vi "ManageQMess.vi"(8 "ErrorIn(No Error)":errorcluster caption="entrée d'erreur (pas d'erreur)", 10 "Message":string, 11 "AppliedMotionDrive.lvclass":refnum<class "AppliedMotionDrive.lvclass">) -> (0 "sortie d'erreur":errorcluster, 3 "AppliedMotionDrive.lvclass Out":refnum<class "AppliedMotionDrive.lvclass">)   [LabVIEW 2019, in "AppliedMotionDrive.lvclass"]
uses:
  AppliedMotionDrive.lvclass
  BaseDevice/ClassQueueMess.ctl
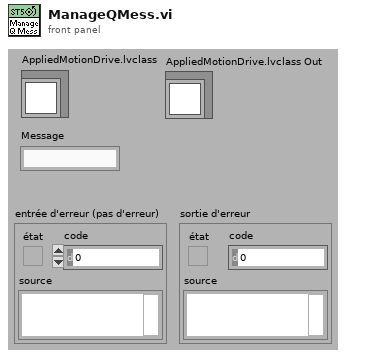
[diagram p1: front panel]
types:
  T1 = typedef "ClassQueueMess.ctl" = u16
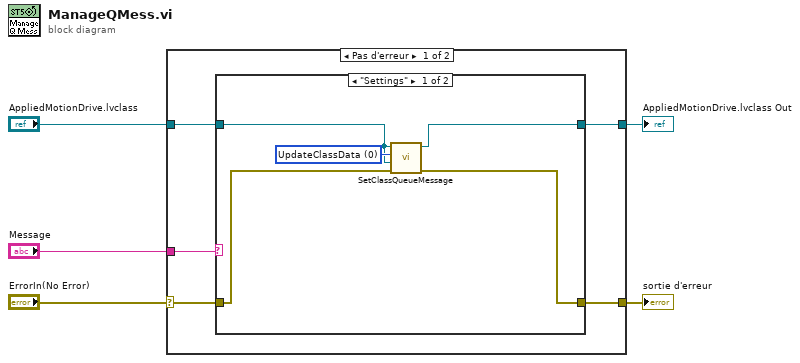
[diagram p0: block diagram]
diagram:
  n1 = case shown="Pas d'erreur" "ErrorIn(No Error)" {
    selector: "ErrorIn(No Error)" -> [w8 w18]
    tunnel: [w9 w18] -> w4
    tunnel: "Message" -> [w10 _]
    tunnel: [w7 w19] -> w2
    tunnel: "AppliedMotionDrive.lvclass" -> [w6 w19]
    frame No Error {
      n2 = case shown="\"Settings\"" w10 {
        tunnel: [w13 w17] -> w9
        tunnel: w8 -> [w14 w17]
        tunnel: [w15 w16] -> w7
        tunnel: w6 -> [w11 w16]
        frame "Settings" {
          w12 = T1 0 items=["UpdateClassData", "UpdateMainClass", "UpdateDataBind", "ReInitDevice", "Custom", "ClosePan"] ("Menu déroulant")
          n3 = call-dynamic "SetClassQueueMessage.vi"("ErrorIn(No Error)"=w14, "Data"=w11, "Menu déroulant"=w12, "AppliedMotionDrive.lvclass"=w11) -> ("sortie d'erreur"=w13:errorcluster, "AppliedMotionDrive.lvclass Out"=w15:refnum<class "AppliedMotionDrive.lvclass">)  [unwired: 6 in]
        }
        frame "", Default {
        }
      }
    }
    frame Error {
    }
  }
  "sortie d'erreur" <- w4
  "AppliedMotionDrive.lvclass Out" <- w2
